vi "read_attributes.vi"(8 "error in (no error)":errorcluster, 11 "RidgeClassifierCV in":refnum<class "RidgeClassifierCV.lvclass">) -> (0 "error out":errorcluster, 2 "attributes":T1, 3 "RidgeClassifierCV out":refnum<class "RidgeClassifierCV.lvclass">)   [LabVIEW 2020, in "RidgeClassifierCV.lvclass"]
uses:
  RidgeClassifierCV.lvclass
  Controls/ridge_classifier_cv_attributes.ctl
  RidgeClassifierCV.lvclass/RidgeClassifierCV.ctl
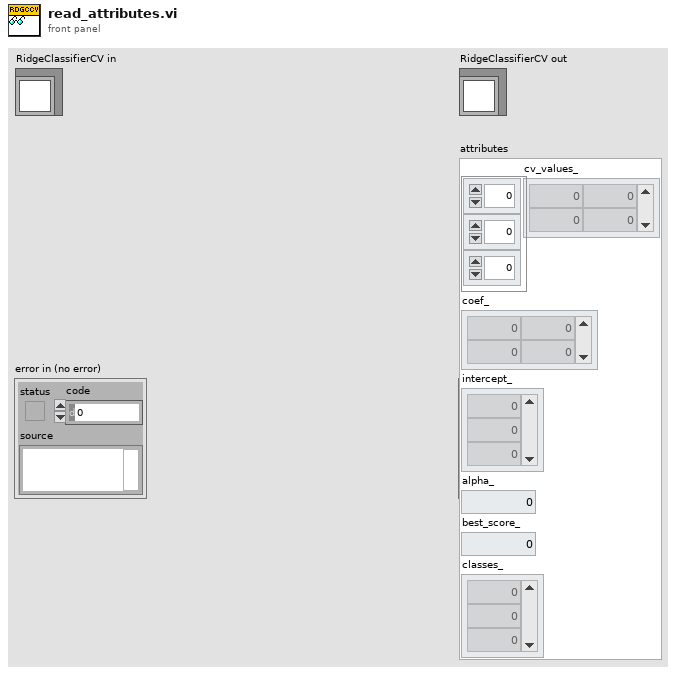
[diagram p1: front panel]
types:
  T1 = typedef "ridge_classifier_cv_attributes.ctl" = cluster{"cv_values_":dbl[][][], "coef_":dbl[][], "intercept_":dbl[], "alpha_":dbl, "best_score_":dbl, "classes_":dbl[]}
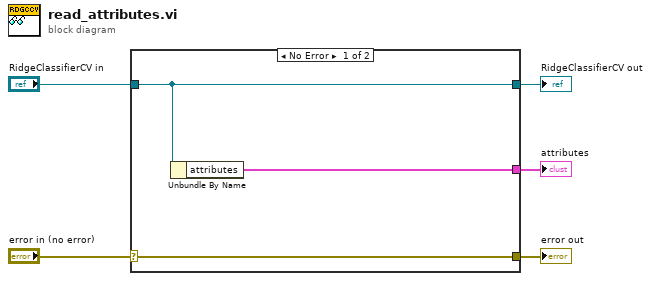
[diagram p0: block diagram]
diagram:
  n1 = case shown="No Error" "error in (no error)" {
    selector: "error in (no error)" -> [w8 w9]
    tunnel: [w8 w9] -> w4
    tunnel: [w7 w10] -> w2
    tunnel: "RidgeClassifierCV in" -> [w7 w10]
    tunnel: [w6 _] -> w1
    frame No Error {
      n2 = Unbundle By Name(w7) -> ("attributes"=w6:T1)
    }
    frame Error {
    }
  }
  "error out" <- w4
  "RidgeClassifierCV out" <- w2
  "attributes" <- w1
